vi "Close.vi"(8 "error in (no error)":errorcluster, 11 "Thorlabs_PM100D in":refnum<class "Thorlabs_PM100D.lvclass">) -> (0 "error out":errorcluster, 3 "Thorlabs_PM100D out":refnum<class "Thorlabs_PM100D.lvclass">)   [LabVIEW 2020, in "Thorlabs_PM100D.lvclass"]
uses:
  <instrlib>/Classes/Powermeter/Thorlabs_PM100D/Thorlabs_PM100D.lvclass
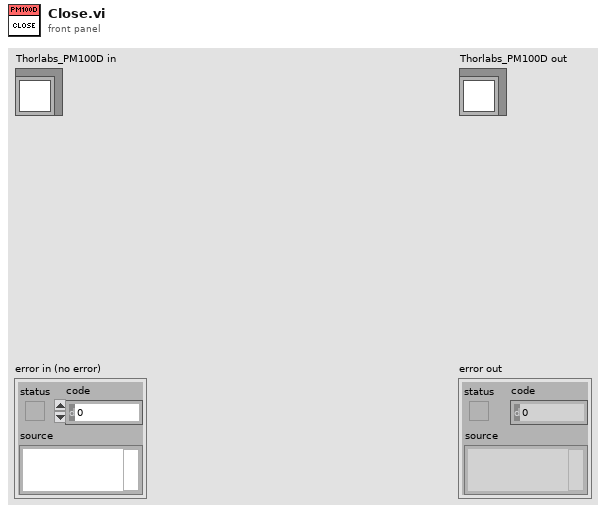
[diagram p1: front panel]
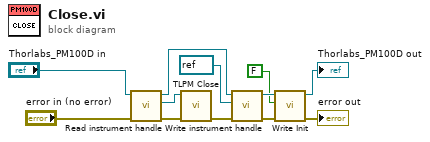
[diagram p0: block diagram]
diagram:
  n1 = call-dynamic "Read instrument handle.vi"("error in (no error)"="error in (no error)", "Thorlabs_PM100D in"="Thorlabs_PM100D in") -> ("error out"=w10:errorcluster, "instrument handle"=w9:refnum<visa-resource-name>, "Thorlabs_PM100D out"=w1:refnum<class "Thorlabs_PM100D.lvclass">)  [unwired: 7 in]
  n2 = call <instrlib>:"TLPM Close.vi"("error in (no error)"=w10, "instrument handle"=w9) -> ("error out"=w8:errorcluster)  [unwired: 9 in]
  n3 = call-dynamic "Write instrument handle.vi"("error in (no error)"=w8, "instrument handle"=refnum<visa-resource-name> refnum, "Thorlabs_PM100D in"=w1) -> ("error out"=w4:errorcluster, "Thorlabs_PM100D out"=w6:refnum<class "Thorlabs_PM100D.lvclass">)  [unwired: 7 in]
  n4 = call-dynamic "Write Init.vi"("error in (no error)"=w4, "Init"=FALSE, "Thorlabs_PM100D in"=w6) -> ("error out"=→"error out":errorcluster, "Thorlabs_PM100D out"=→"Thorlabs_PM100D out":refnum<class "Thorlabs_PM100D.lvclass">)  [unwired: 7 in]
